vi "ERD Read Test Template (String_Enum).vi"(0 "GEA2 Reference In":refnum<k24>, 5 "Standalone?":bool, 7 "Enum":enum16{""}(ring), 11 "Error In":errorcluster) -> (4 "GEA2 Reference Out":refnum<k24>, 6 "Pass/Fail?":bool, 15 "Error Out":errorcluster)   [LabVIEW 2016, in "2015 VA Washer.lvlib"]
uses:
  Projects/2015 VA Washer.lvlib
  C:/Automation/DLLs/PC Dot Net/GeaCommunication.dll
  Common/LabVIEW GEA2 Toolkit/LabVIEW_GEA2_Toolkit.lvlibp/type defs/Source_Destination.ctl
  Common/LabVIEW GEA2 Toolkit/LabVIEW_GEA2_Toolkit.lvlibp/type defs/ERD Read Data In.ctl
  Common/LabVIEW GEA2 Toolkit/LabVIEW_GEA2_Toolkit.lvlibp/type defs/Data Type.ctl
  Common/LabVIEW GEA2 Toolkit/LabVIEW_GEA2_Toolkit.lvlibp
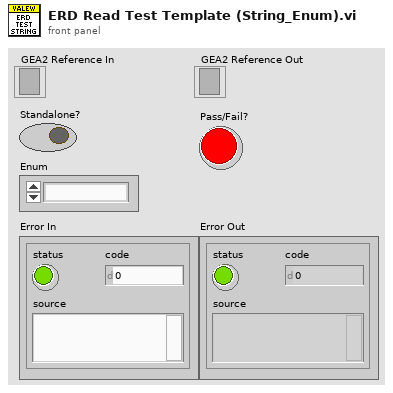
[diagram p1: front panel]
types:
  T1 = typedef "LabVIEW_GEA2_Toolkit.lvlibp/ERD Read Data In.ctl" = cluster{"ERD Number":u16, "Data Type":T2}
  T2 = typedef "LabVIEW_GEA2_Toolkit.lvlibp/Data Type.ctl" = enum16{"string", "boolean", "uint8_t", "uint16_t", "uint32_t", "uint64_t", "int8_t", "int16_t", "int32_t", "int64_t"}
  T3 = typedef "LabVIEW_GEA2_Toolkit.lvlibp/Source_Destination.ctl" = cluster{"Source":u8, "Destination":u8}
  T4 = typedef "LabVIEW_GEA2_Toolkit.lvlibp/ERD Read Data Out.ctl" = cluster{"ERD Number":u16, "Data":string}
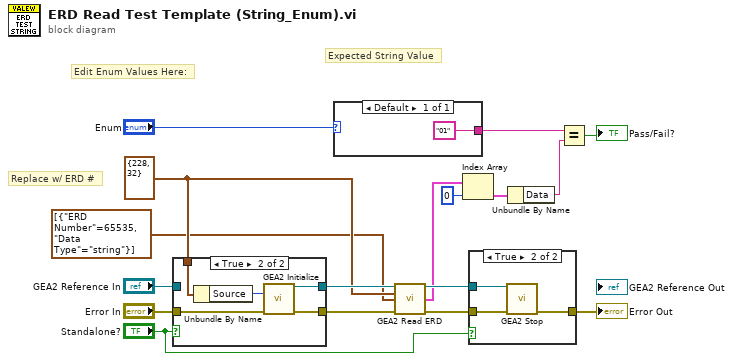
[diagram p0: block diagram]
diagram:
  w9 = T3 {"Source"=228, "Destination"=32} ("GEA Inputs")
  # "Expected String Value"
  # "Edit Enum Values Here:"
  # "Replace w/ ERD #"
  n1 = case shown="True" "Standalone?" {
    tunnel: "Error In" -> [w18 w24]
    tunnel: [w18 w23] -> w13
    tunnel: "GEA2 Reference In" -> [w19 _]
    tunnel: [w19 w22] -> w11
    tunnel: w9 -> [_ w20]
    frame False {
    }
    frame True {
      n2 = Unbundle By Name(w20) -> ("Source"=w21:u8)
      n3 = call "GEA2 Initialize.vi"("Source Address"=w21, "error in"=w24) -> ("GEA2 Reference Out"=w22:refnum<k24>, "error out"=w23:errorcluster)  [unwired: 11 in, 1 out]
    }
  }
  n4 = case shown="Default" "Enum" {
    tunnel: ["01"] -> w2
    frame Default {
    }
  }
  n5 = call "GEA2 Read ERD.vi"("GEA2 Reference In"=w11, "GEA Inputs"=w9, "Read ERD List"=T1[] [{"ERD Number"=65535, "Data Type"=enum."string"}], "Error In"=w13) -> ("GEA2 Reference Out"=w10:refnum<k24>, "ERD Data Out"=w7:T4[], "Error Out"=w12:errorcluster)  [unwired: 8 in, 1 out]
  n6 = Index Array(array=w7, index=0) -> (element=w5:T4)
  n7 = case shown="True" "Standalone?" {
    tunnel: [w26 w29] -> w15
    tunnel: w12 -> [w26 w28]
    tunnel: w10 -> [_ w27]
    frame False {
    }
    frame True {
      n8 = call "GEA2 Stop.vi"("GEA2 Reference In"=w27, "Error In"=w28) -> ("Error Out"=w29:errorcluster)  [unwired: 13 in]
    }
  }
  "Error Out" <- w15
  n9 = Unbundle By Name(w5) -> ("Data"=w4:string)
  n10 = Equal?(x=w2, y=w4) -> (x = y?=→"Pass/Fail?":bool)
